vi "DialogCfg.vi"(8 "error in (no error)":errorcluster, 10 "VXMCfg in":refnum<class "VXMCfg.lvclass">=refnum, 11 "aparCfg in":refnum<class "aparCfg.lvclass">) -> (0 "error out":errorcluster, 1 "Cancelled?":bool, 2 "VXMCfg out":refnum<class "VXMCfg.lvclass">, 3 "aparCfg out":refnum<class "aparCfg.lvclass">, 4 "Motion Restart":enum16{"NoOp", "Start", "Stop"}(ring))   [LabVIEW 2018, in "aparCfg.lvclass"]
uses:
  aparCfg.lvclass
  ArrayController/ACConfig.ctl
  VXMCfg/VXMCfg.lvclass
  aparCfg.lvclass/aparCfg.ctl
panel:
  in  "VXM-2 Serial Port Sub-syst.3":cluster{"Addr":string, "Enable":bool}
  in  "VXM-4 Serial Port Sub-syst.2":cluster{"Addr":string, "Enable":bool}
  in  "VXM-3 Serial Port Sub-syst.1":cluster{"Addr":string, "Enable":bool}
  in  "apar properties":T2={"N5222AConfig"={"ResourceName"="", "Enable"=FALSE, "Channel"=1, "CalFileName"="", "MeasName"="", "TempDatFile"="", "Power, dBm"=-30.0, "Number of Points"=0, "Start Freq, Hz"=5000000000.0, "Stop Freq, Hz"=6000000000.0, "NumAverages"=201, "Sweep Type"=0}, "ACConfig"={"Board 1 alias"="192.168.1.110", "Board 1 Enable"=FALSE, "Board 2 alias"="192.168.1.110", "Board 2 Enable"=FALSE}, "DataLogConfig"={"Data Directory Path"=path ""}} {"N5222AConfig"."Sweep Type" items=["Linear Frequency", "Log Frequency", "Power Sweep", "CW Time"]; "N5222AConfig"."Stop Freq, Hz" format="%_3p"; "N5222AConfig"."Start Freq, Hz" format="%_3p"; "N5222AConfig"."Number of Points" items=["2"=2, "3"=3, "11"=11, "21"=21, "51"=51, "101"=101, "201"=201, "401"=401, "801"=801, "1601"=1601, "3201"=3201, "6401"=6401, "12801"=12801, "16001"=16001, "20001"=20001]}
  in  "Cancel":bool
  in  "OK":bool
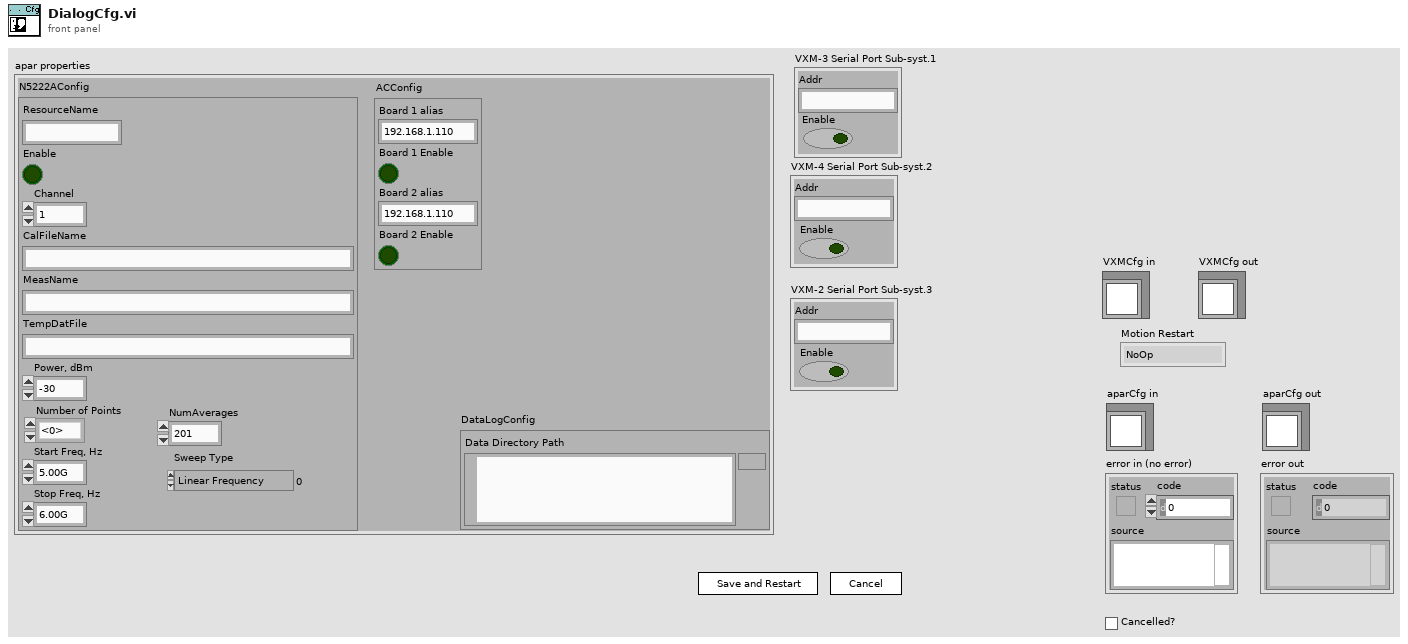
[diagram p1: front panel]
types:
  T1 = typedef "ACConfig.ctl" = cluster{"Board 1 alias":string, "Board 1 Enable":bool, "Board 2 alias":string, "Board 2 Enable":bool}
  T2 = cluster{"N5222AConfig":cluster{"ResourceName":string, "Enable":bool, "Channel":i32, "CalFileName":string, "MeasName":string, "TempDatFile":string, "Power, dBm":dbl, "Number of Points":u16, "Start Freq, Hz":dbl, "Stop Freq, Hz":dbl, "NumAverages":i32, "Sweep Type":i32}, "ACConfig":T1, "DataLogConfig":cluster{"Data Directory Path":path}}
  T3 = typedef "aparCfg.lvclass/aparConfig.ctl" = cluster{"N5222AConfig":T4, "ACConfig":T1, "DataLogConfig":T5}
  T4 = typedef "N5222AConfig.ctl" = cluster{"ResourceName":string, "Enable":bool, "Channel":i32, "CalFileName":string, "MeasName":string, "TempDatFile":string, "Power, dBm":dbl, "NumPoints":i32, "Start Freq, Hz":dbl, "Stop Freq, Hz":dbl, "NumAverages":i32, "Sweep Type":i32}
  T5 = typedef "DataLogConfig.ctl" = cluster{"FilePath":path}
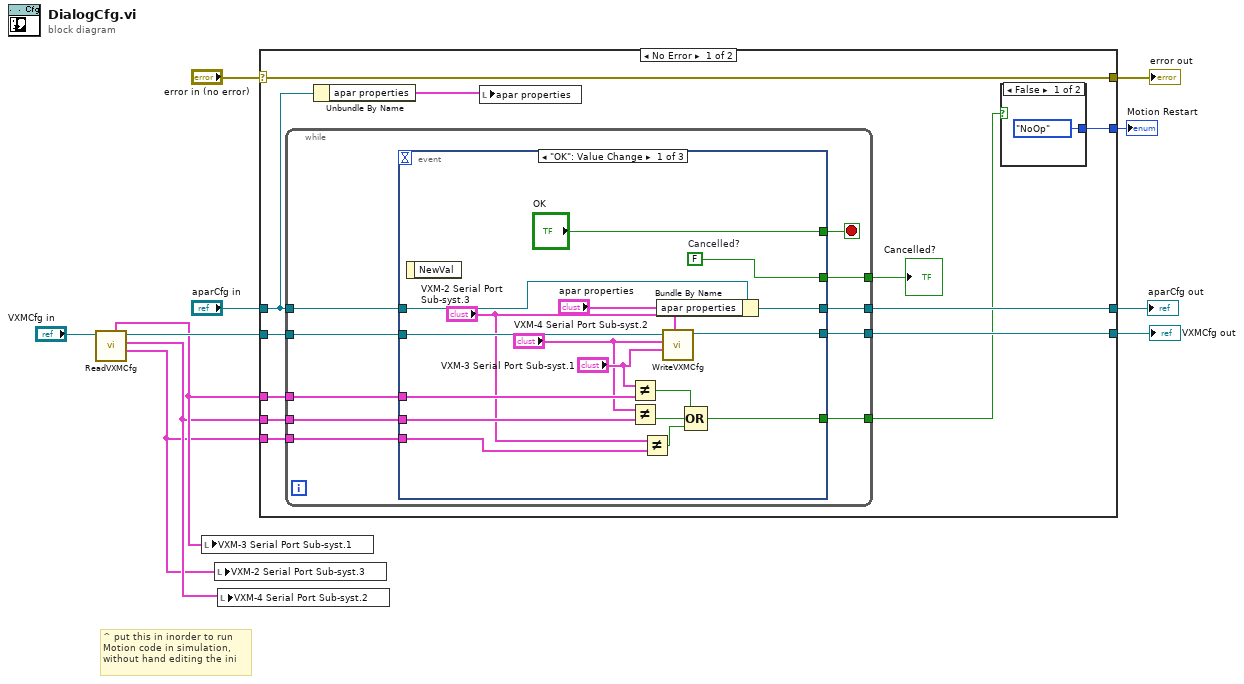
[diagram p0: block diagram]
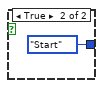
[diagram p2: hidden frame]
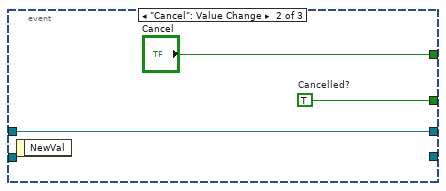
[diagram p3: hidden frame]
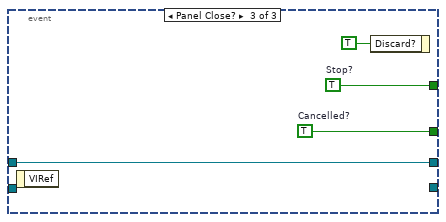
[diagram p4: hidden frame]
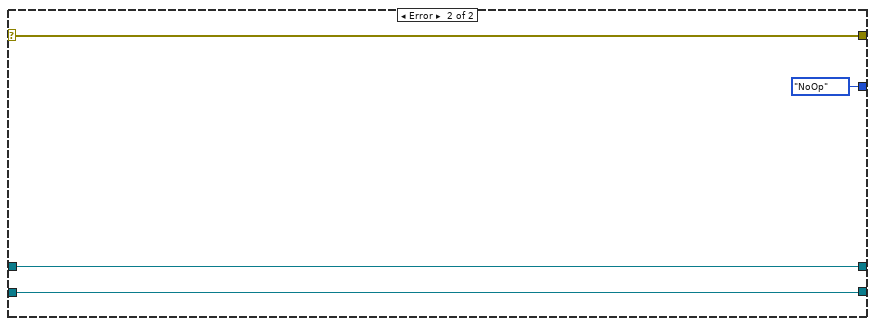
[diagram p5: hidden frame]
diagram:
  # "^ put this in inorder to run\nMotion code in simulation,\nwithout hand editing the ini"
  n1 = call "ReadVXMCfg.vi"("VXMCfg in"="VXMCfg in") -> ("VXM Properties.Serial Port 3"=w1:cluster{"Addr":string, "Enable":bool}, "VXM Properties.Serial Port 2"=w2:cluster{"Addr":string, "Enable":bool}, "VXMCfg out"=w4:refnum<class "VXMCfg.lvclass">, "VXM Properties.Serial Port"=w3:cluster{"Addr":string, "Enable":bool})  [unwired: 6 in, 1 out]
  n2 = local write "VXM-3 Serial Port Sub-syst.1"(w3) -> ()
  n3 = local write "VXM-2 Serial Port Sub-syst.3"(w1) -> ()
  n4 = local write "VXM-4 Serial Port Sub-syst.2"(w2) -> ()
  n5 = case shown="No Error" "error in (no error)" {
    selector: "error in (no error)" -> [w23 w63]
    tunnel: [w23 w63] -> w9
    tunnel: [w20 w62] -> w8
    tunnel: "aparCfg in" -> [w21 w62]
    tunnel: [w18 enum16{"NoOp", "Start", "Stop"}."NoOp"] -> w7
    tunnel: w4 -> [w17 w60]
    tunnel: [w16 w60] -> w6
    tunnel: w3 -> [w15 _]
    tunnel: w2 -> [w14 _]
    tunnel: w1 -> [w13 _]
    frame No Error {
      n6 = while {
        tunnel: [w34] -> w22
        tunnel: w21 -> [w33]
        tunnel: [w32] -> w20
        tunnel: w17 -> [w31]
        tunnel: [w30] -> w16
        tunnel: w15 -> [w29]
        tunnel: w14 -> [w28]
        tunnel: w13 -> [w27]
        tunnel: [w26] -> w12
        stop <- w35 stop-if-true
        n7 = event shown="[0] \"OK\": Value Change" {
          selector: _ -> [_ _ _]
          dyn-events: _ -> [_ _ _]
          timeout: _ -> [_ _ _]
          tunnel: ["OK" "Cancel" w58] -> w35
          tunnel: [w52 w55 w57] -> w34
          tunnel: [w50 w53 w56] -> w32
          tunnel: w33 -> [w49 w53 w56]
          tunnel: w31 -> [w47 _ _]
          tunnel: [w46 _ _] -> w30
          tunnel: w29 -> [w44 _ _]
          tunnel: w28 -> [w42 _ _]
          tunnel: w27 -> [w40 _ _]
          tunnel: [w36 _ _] -> w26
          event "OK": Value Change {
            w52 = FALSE  # Cancelled?
            n8 = event-data() -> ()  [unwired: 1 in, 1 out]
            n9 = Not Equal?(x="VXM-3 Serial Port Sub-syst.1", y=w44) -> (x != y?=w39:bool)
            n10 = Not Equal?(x="VXM-4 Serial Port Sub-syst.2", y=w42) -> (x != y?=w37:bool)
            n11 = Not Equal?(x="VXM-2 Serial Port Sub-syst.3", y=w40) -> (x != y?=w38:bool)
            n12 = Bundle By Name(cluster=w49, "apar properties"="apar properties") -> (w50:refnum<class "aparCfg.lvclass">)
            n13 = call "WriteVXMCfg.vi"("VXM Properties.Serial Port 3"="VXM-2 Serial Port Sub-syst.3", "VXM Properties.Serial Port"="VXM-3 Serial Port Sub-syst.1", "VXM Properties.Serial Port 2"="VXM-4 Serial Port Sub-syst.2", "VXMCfg in"=w47) -> ("VXMCfg out"=w46:refnum<class "VXMCfg.lvclass">)  [unwired: 6 in, 1 out]
            n14 = Compound Arithmetic op=OR(w39, w37, w38) -> (w36:bool)
          }
          event "Cancel": Value Change {
            w55 = TRUE  # Cancelled?
            n15 = event-data() -> ()  [unwired: 1 in, 1 out]
          }
          event Panel Close? {
            w57 = TRUE  # Cancelled?
            w58 = TRUE  # Stop?
            n16 = event-data() -> ()  [unwired: 1 in, 1 out]
            n17 = event-data("Discard?"=TRUE) -> ()  [unwired: 1 in, 1 out]
          }
        }
      }
      "Cancelled?" <- w22
      n18 = Unbundle By Name(w21) -> ("apar properties"=w19:T3)
      n19 = local write "apar properties"(w19) -> ()
      n20 = case shown="False" w12 {
        tunnel: [enum16{"NoOp", "Start", "Stop"}."NoOp" enum16{"NoOp", "Start", "Stop"}."Start"] -> w18
        frame False {
        }
        frame True {
        }
      }
    }
    frame Error {
    }
  }
  "error out" <- w9
  "aparCfg out" <- w8
  "Motion Restart" <- w7
  "VXMCfg out" <- w6
